vi "Read WriteUrgent.vi"(8 "error in (no error)":errorcluster, 11 "ICPCON ET Data Model in":refnum<class "ICPCON ET Data Model.lvclass">) -> (0 "error out":errorcluster, 2 "WriteUrgent":refnum<notifier>, 3 "ICPCON ET Data Model out":refnum<class "ICPCON ET Data Model.lvclass">)   [LabVIEW 2021, in "ICPCON ET Data Model.lvclass"]
uses:
  ICPCON ET Data Model.lvclass
  ICPCON ET Data Model.lvclass/ICPCON ET Data Model.ctl
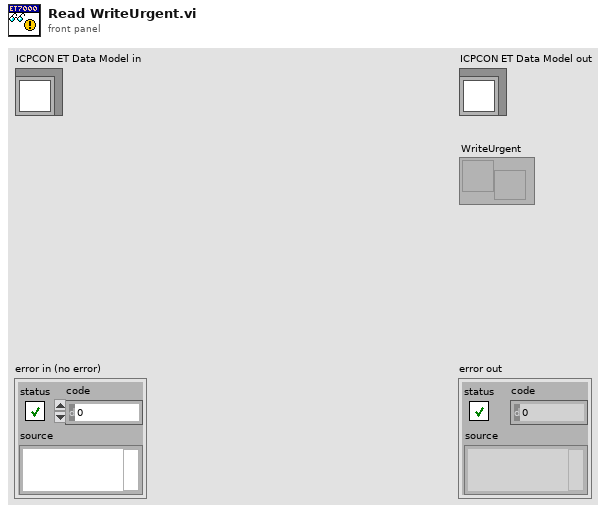
[diagram p1: front panel]
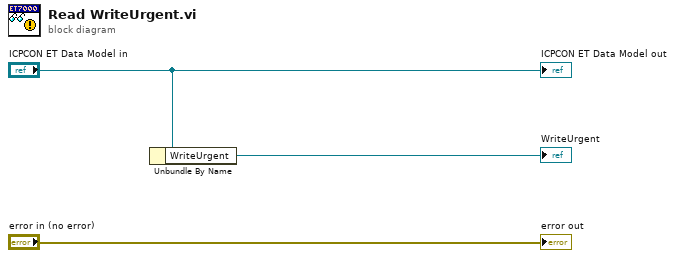
[diagram p0: block diagram]
diagram:
  n1 = Unbundle By Name("ICPCON ET Data Model in") -> ("WriteUrgent"=→"WriteUrgent":refnum<notifier>)
  "error out" <- "error in (no error)"
  "ICPCON ET Data Model out" <- "ICPCON ET Data Model in"
